vi "Get Name and Path.vi"(8 "error in (no error)":errorcluster, 11 "Application Controller in":refnum<class "Application Controller.lvclass">) -> (0 "error out":errorcluster, 1 "Name":string, 2 "Application folder":path, 3 "Application Controller out":refnum<class "Application Controller.lvclass">, 4 "Start-up configuration path":path)   [LabVIEW 2016, in "Application Controller.lvclass"]
uses:
  Application Controller.lvclass
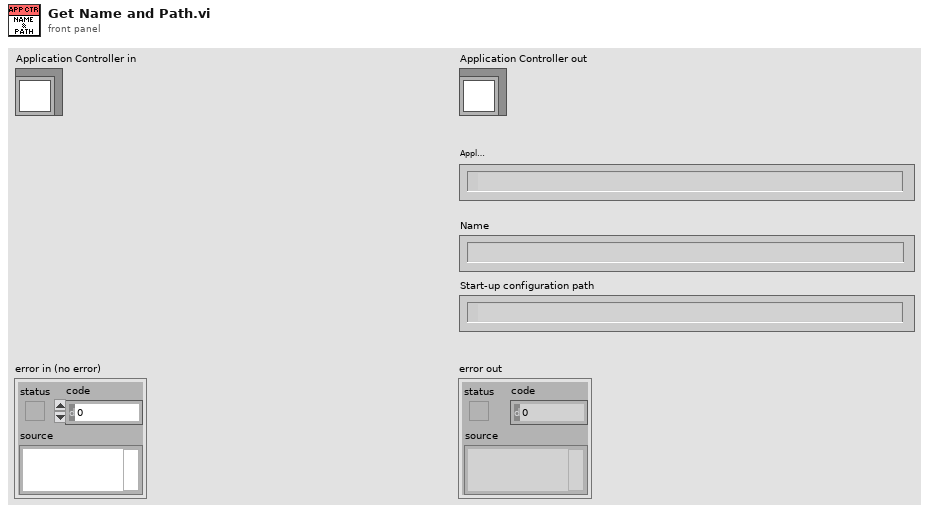
[diagram p1: front panel]
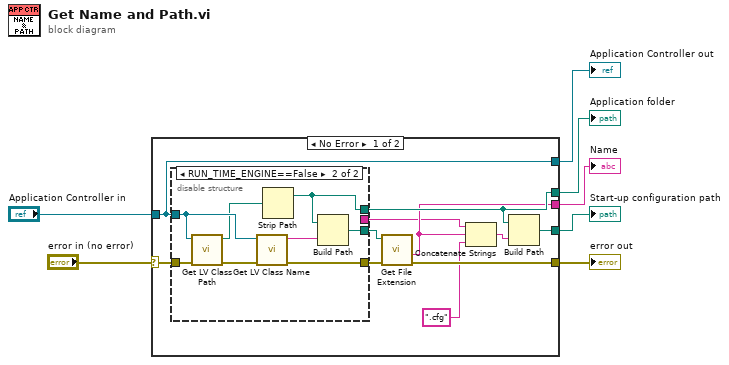
[diagram p0: block diagram]
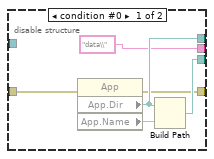
[diagram p2: hidden frame]
diagram:
  n1 = case shown="No Error" "error in (no error)" {
    selector: "error in (no error)" -> [w17 w34]
    tunnel: [w15 w34] -> w6
    tunnel: [w18 w33] -> w4
    tunnel: "Application Controller in" -> [w18 w33]
    tunnel: [w12 _] -> w3
    tunnel: [w13 _] -> w2
    tunnel: [w9 _] -> w1
    frame No Error {
      n2 = disable-structure shown="RUN_TIME_ENGINE==False" {
        disable-tunnel: [w23 w25] -> w13
        disable-tunnel: w18 -> [_ w31]
        disable-tunnel: w17 -> [w22 w32]
        disable-tunnel: [w20 w29] -> w16
        disable-tunnel: [w21 w26] -> w14
        disable-tunnel: ["data\\" ("string") _] -> w8
        frame condition #0 {
          n3 = property class="App"(error in=w22) -> (error out=w20:errorcluster, "App.Dir"=w23:path, "App.Name"=w24:string)  [unwired: 1 in, 1 out]
          n4 = Build Path(base path=w23, name or relative path=w24) -> (appended path=w21:path)
        }
        frame condition #1 (active) {
          n5 = call <vilib>:"Get LV Class Path.vi"("error in (no error)"=w32, "object"=w31) -> ("error out"=w30:errorcluster, "class path"=w28:path)  [unwired: 8 in]
          n6 = call <vilib>:"Get LV Class Name.vi"("error in (no error)"=w30, "object"=w31) -> ("error out"=w29:errorcluster, "class name"=w27:string)  [unwired: 8 in]
          n7 = Strip Path(path=w28) -> (stripped path=w25:path)  [unwired: 1 out]
          n8 = Build Path(base path=w25, name or relative path=w27) -> (appended path=w26:path)
        }
      }
      n9 = call <vilib>:"Get File Extension.vi"("error in (no error)"=w16, "file"=w14) -> ("error out"=w15:errorcluster, "filename without extension"=w12:string)  [unwired: 5 in, 3 out]
      n10 = Concatenate Strings(w8, w12, ".cfg") -> (w10:string)
      n11 = Build Path(base path=w13, name or relative path=w10) -> (appended path=w9:path)
    }
    frame Error {
    }
  }
  "error out" <- w6
  "Application Controller out" <- w4
  "Name" <- w3
  "Application folder" <- w2
  "Start-up configuration path" <- w1
